vi "Log Warnings.vi"(8 "Error In":errorcluster, 10 "Weather Data":T1, 11 "file ref in":refnum<file>) -> (0 "Error Out":errorcluster, 3 "file ref out":refnum<file>)   [LabVIEW 2019]
uses:
  Weather Data.ctl
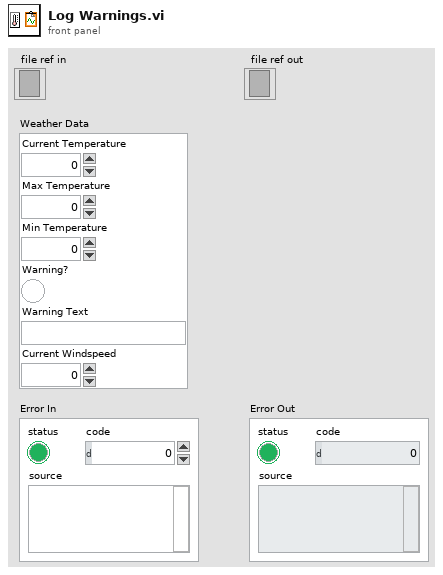
[diagram p1: front panel]
types:
  T1 = typedef "Weather Data.ctl" = cluster{"Current Temperature":dbl, "Max Temperature":dbl, "Min Temperature":dbl, "Warning?":bool, "Warning Text":string, "Current Windspeed":dbl}
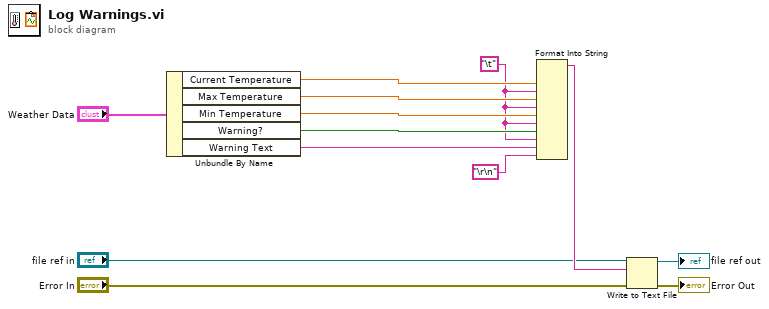
[diagram p0: block diagram]
diagram:
  w9 = "\t"
  n1 = Unbundle By Name("Weather Data") -> ("Current Temperature"=w13:dbl, "Max Temperature"=w12:dbl, "Min Temperature"=w11:dbl, "Warning?"=w10:bool, "Warning Text"=w8:string)
  n2 = Format Into String(w13, w9, w12, w9, w11, w9, w10, w9, w8, "\r\n") -> (resulting string=w6:string)  [unwired: 3 in, 1 out]
  n3 = Write to Text File(file (use dialog)="file ref in", text=w6, error in="Error In") -> (refnum out=→"file ref out":refnum<file>, error out=→"Error Out":errorcluster)  [unwired: 1 in, 1 out]
